vi "write_date_attributes.vi"(8 "error in (no error)":errorcluster, 11 "HDF5 Ref":T1) -> (0 "error out":errorcluster, 3 "HDF5 Ref out":T1)   [LabVIEW 2015, in "hdf5_photon_record_log.lvclass"]
uses:
  hdf5_photon_record_log.lvclass
  <vilib>/UPVI/lvhdf5/library.llb/HDF5 Ref.ctl
  <vilib>/UPVI/lvhdf5/attribute.llb/Simple H5Awrite (Variant).vi
  <vilib>/UPVI/lvhdf5/attribute.llb/LVH5A Operation.ctl
  <vilib>/UPVI/lvhdf5/attribute.llb/Simple H5Awrite.xnode
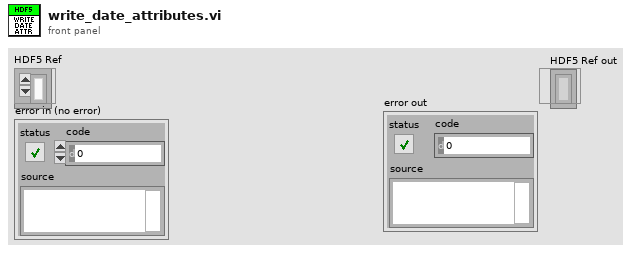
[diagram p1: front panel]
types:
  T1 = typedef "HDF5 Ref.ctl" = refnum<k1>
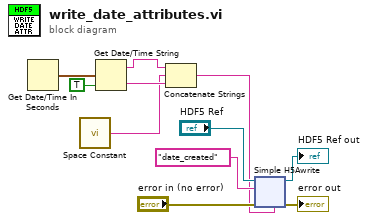
[diagram p0: block diagram]
diagram:
  n1 = Get Date/Time In Seconds() -> (seconds since 1Jan1904=w6:timestamp)
  n2 = call <vilib>:"Space Constant.vi"() -> ("String"=w1:string)
  n3 = Get Date/Time String(seconds (now)=w6, want seconds? (F)=TRUE) -> (date string=w2:string, time string=w4:string)  [unwired: 1 in]
  n4 = Concatenate Strings(w2, w1, w4) -> (w3:string)
  n5 = xnode "Simple H5Awrite"("HDF5 Ref"="HDF5 Ref", "Name"="date_created", "error in (no error)"="error in (no error)", "Value"=w3) -> ("HDF5 Ref out"=→"HDF5 Ref out":T1, "error out"=→"error out":errorcluster)  [unwired: 1 in]
